vi "BG-corr-eventSD.vi"(1 "Single":bool, 2 "cluster in":T1={"Kinetics"=[], "Spectrum"=[], "Experiments groups"=[], "GRAPH EXPERIMENTAL DATA"=[], "error out"={"status"=FALSE, "code"=0, "source"=""}, "group"=0, "exp selected"=0, "# exp"=0, "kinetics plot names"=[], "spectra plot names"=[], "FromToWave"={"FromWave"=0.0, "ToWave"=0.0}, "Laser shutter task"="", "Accelerator task"="", "Motor task"="", "GRAPH EXPERIMENTAL DATA ref"=refnum, "timedelays"=[0.0, 0.0, 0.0, 0.0, 0.0, 0.0, 0.0, 0.06019061100911815, 0.0521779104562645, 0.045231877429679615, 0.03921051490799832, 0.033990728811568754, 0.029465811603150715, 0.025543260876973825, 0.02214288834180205, 0.01919518054014414, 0.016639877791965713, 0.014424742312398925, 0.012504490320209958, 0.010839866306230088, 0.009396840537117498, 0.008145913389103785, 0.00706151229029317, 0.006121468943269439, 0.005306566140927374, 0.004600144911132549, 0.003987763959109073, 0.0034569044455719407, 0.00299671406541447, 0.0025977851951783253, 0.0022519625739982996, 0.00195217658646366, 0.0016922987392150965, 0.0014670163768006634, 0.0012717240756200802, 0.0011024294957352762, 0.0009556717658856477, 0.0008284507332614981, 0.0007181656316962257, 0.0006225619144775864, 0.0005396851648867825, 0.00046784114226338394, 0.0004055611468220084, 0.0003515719951773376, 0.00030476999279031153, 0.00026419837125694315, 0.00022902772919263772, 0.0001985390768670671, 0.0001721091379728629, 0.00014919760805372974, 0.00012933610911736794], "wavelengths"=[0.0, 0.0, 0.0, 0.0, 0.0, 0.0, 0.0, 0.06019061100911815, 0.0521779104562645, 0.045231877429679615, 0.03921051490799832, 0.033990728811568754, 0.029465811603150715, 0.025543260876973825, 0.02214288834180205, 0.01919518054014414, 0.016639877791965713, 0.014424742312398925, 0.012504490320209958, 0.010839866306230088, 0.009396840537117498, 0.008145913389103785, 0.00706151229029317, 0.006121468943269439, 0.005306566140927374, 0.004600144911132549, 0.003987763959109073, 0.0034569044455719407, 0.00299671406541447, 0.0025977851951783253, 0.0022519625739982996, 0.00195217658646366, 0.0016922987392150965, 0.0014670163768006634, 0.0012717240756200802, 0.0011024294957352762, 0.0009556717658856477, 0.0008284507332614981, 0.0007181656316962257, 0.0006225619144775864, 0.0005396851648867825, 0.00046784114226338394, 0.0004055611468220084, 0.0003515719951773376, 0.00030476999279031153, 0.00026419837125694315, 0.00022902772919263772, 0.0001985390768670671, 0.0001721091379728629, 0.00014919760805372974, 0.00012933610911736794], "Experiment"=refnum, "Commentaires exp"=refnum, "FromToDelay"={"FromDelay"=0.0, "ToDelay"=0.0}}, 3 "Update graphs of exp":refnum<user-event>, 4 "def pixel lower":dbl, 5 "def pixel upper":dbl) -> (0 "cluster out":T1={"Kinetics"=[], "Spectrum"=[], "Experiments groups"=[], "GRAPH EXPERIMENTAL DATA"=[], "error out"={"status"=FALSE, "code"=0, "source"=""}, "group"=0, "exp selected"=0, "# exp"=0, "kinetics plot names"=[], "spectra plot names"=[], "FromToWave"={"FromWave"=0.0, "ToWave"=0.0}, "Laser shutter task"="", "Accelerator task"="", "Motor task"="", "GRAPH EXPERIMENTAL DATA ref"=refnum, "timedelays"=[0.0, 0.0, 0.0, 0.0, 0.0, 0.0, 0.0, 0.06019061100911815, 0.0521779104562645, 0.045231877429679615, 0.03921051490799832, 0.033990728811568754, 0.029465811603150715, 0.025543260876973825, 0.02214288834180205, 0.01919518054014414, 0.016639877791965713, 0.014424742312398925, 0.012504490320209958, 0.010839866306230088, 0.009396840537117498, 0.008145913389103785, 0.00706151229029317, 0.006121468943269439, 0.005306566140927374, 0.004600144911132549, 0.003987763959109073, 0.0034569044455719407, 0.00299671406541447, 0.0025977851951783253, 0.0022519625739982996, 0.00195217658646366, 0.0016922987392150965, 0.0014670163768006634, 0.0012717240756200802, 0.0011024294957352762, 0.0009556717658856477, 0.0008284507332614981, 0.0007181656316962257, 0.0006225619144775864, 0.0005396851648867825, 0.00046784114226338394, 0.0004055611468220084, 0.0003515719951773376, 0.00030476999279031153, 0.00026419837125694315, 0.00022902772919263772, 0.0001985390768670671, 0.0001721091379728629, 0.00014919760805372974, 0.00012933610911736794], "wavelengths"=[0.0, 0.0, 0.0, 0.0, 0.0, 0.0, 0.0, 0.06019061100911815, 0.0521779104562645, 0.045231877429679615, 0.03921051490799832, 0.033990728811568754, 0.029465811603150715, 0.025543260876973825, 0.02214288834180205, 0.01919518054014414, 0.016639877791965713, 0.014424742312398925, 0.012504490320209958, 0.010839866306230088, 0.009396840537117498, 0.008145913389103785, 0.00706151229029317, 0.006121468943269439, 0.005306566140927374, 0.004600144911132549, 0.003987763959109073, 0.0034569044455719407, 0.00299671406541447, 0.0025977851951783253, 0.0022519625739982996, 0.00195217658646366, 0.0016922987392150965, 0.0014670163768006634, 0.0012717240756200802, 0.0011024294957352762, 0.0009556717658856477, 0.0008284507332614981, 0.0007181656316962257, 0.0006225619144775864, 0.0005396851648867825, 0.00046784114226338394, 0.0004055611468220084, 0.0003515719951773376, 0.00030476999279031153, 0.00026419837125694315, 0.00022902772919263772, 0.0001985390768670671, 0.0001721091379728629, 0.00014919760805372974, 0.00012933610911736794], "Experiment"=refnum, "Commentaires exp"=refnum, "FromToDelay"={"FromDelay"=0.0, "ToDelay"=0.0}})   [LabVIEW 2015]
uses:
  controls/control-cluster.ctl
  Classes/Experiments_group.lvclass
types:
  T1 = typedef "control-cluster.ctl" = cluster{"Kinetics":cluster{"timedelay":dbl[], dbl[]}[], "Spectrum":cluster{"Unités abscisse":dbl[], dbl[]}[], "Experiments groups":refnum<class "Experiments_group.lvclass">[], "GRAPH EXPERIMENTAL DATA":dbl[][], "error out":errorcluster, "group":i32, "exp selected":i32, "# exp":i32, "kinetics plot names":string[], "spectra plot names":string[], "FromToWave":cluster{"FromWave":dbl, "ToWave":dbl}, "Laser shutter task":refnum<k21>, "Accelerator task":refnum<k21>, "Motor task":refnum<k21>, "GRAPH EXPERIMENTAL DATA ref":refnum<vi>, "timedelays":dbl[], "wavelengths":dbl[], "Experiment":refnum<vi>, "Commentaires exp":refnum<vi>, "FromToDelay":cluster{"FromDelay":dbl, "ToDelay":dbl}}
  T2 = typedef "mylistbox.ctl" = i32[]
  T3 = cluster{bool, "Item Names":string[], "exp selected":i32}
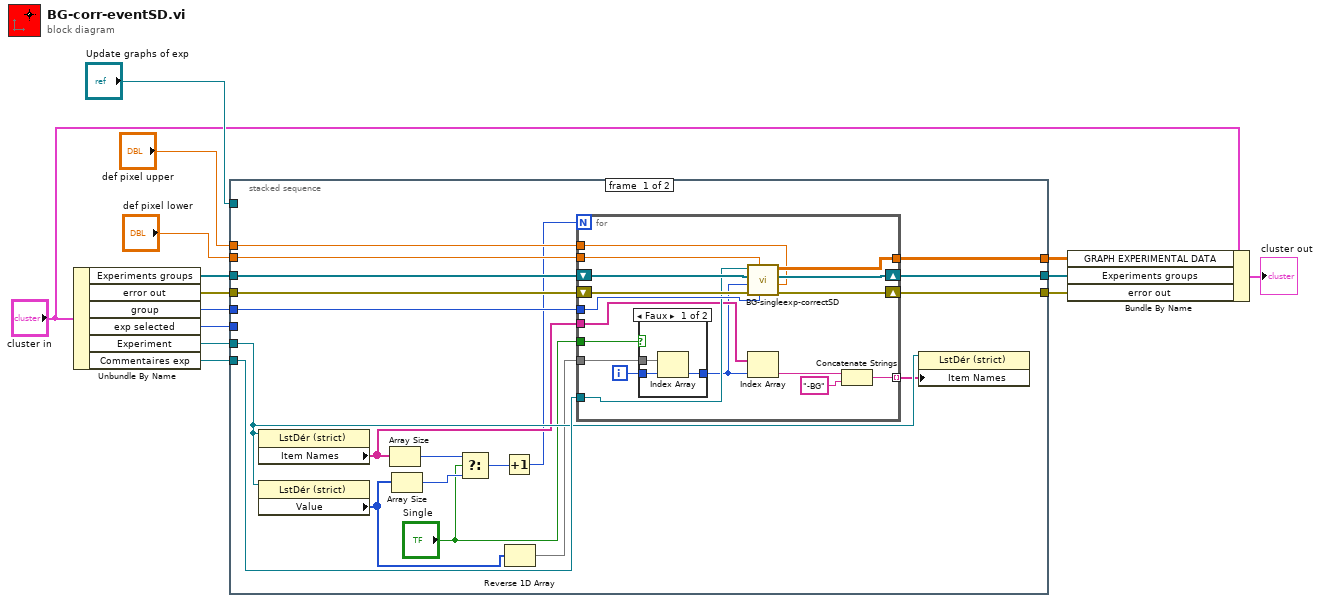
[diagram p0: block diagram]
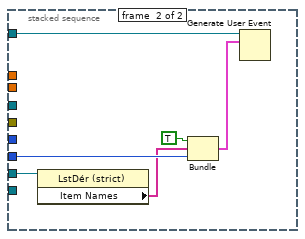
[diagram p3: hidden frame]
diagram:
  n1 = Unbundle By Name("cluster in") -> ("Experiments groups"=w8:refnum<class "Experiments_group.lvclass">[], "error out"=w7:errorcluster, "group"=w4:i32, "exp selected"=w5:i32, "Experiment"=w2:refnum<vi>, "Commentaires exp"=w1:refnum<vi>)
  n2 = stacked-sequence {
    tunnel: [w33 _] -> w9
    tunnel: w5 -> [_ w58]
    tunnel: w8 -> [w31 _]
    tunnel: w7 -> [w32 _]
    tunnel: [w25 _] -> w6
    tunnel: [w30 _] -> w3
    tunnel: "Update graphs of exp" -> [_ w59]
    tunnel: "def pixel lower" -> [w29 _]
    tunnel: "def pixel upper" -> [w28 _]
    tunnel: w4 -> [w27 _]
    tunnel: w1 -> [w26 _]
    tunnel: w2 -> [w24 w57]
    frame #0 {
      n3 = property on="Property Node" class="LstDér (strict)"(reference=w24) -> ("Item Names"=w17:string[])  [unwired: 1 in, 2 out]
      n4 = property class="LstDér (strict)"(reference=w24) -> ("Value"=w20:T2)  [unwired: 1 in, 2 out]
      n5 = Array Size(array=w17) -> (size(s)=w16:i32)
      n6 = Array Size(array=w20) -> (size(s)=w19:i32)
      n7 = Select(t=w16, s="Single", f=w19) -> (s? t:f=w22:i32)
      n8 = Increment(x=w22) -> (x+1=w15:i32)
      n9 = Reverse 1D Array(array=w20) -> (reversed array=w21:T2)
      n10 = for {
        N: w15 -> [_]
        tunnel: [w47] -> w30
        tunnel: w29 -> [w46]
        tunnel: w28 -> [w45]
        tunnel: w27 -> [w44]
        tunnel: w26 -> [w43]
        shift-right: [w42] -> w25
        shift-left: w32 -> [w49]
        tunnel: w21 -> [w35]
        tunnel: w17 -> [w39]
        tunnel: [w38] -> w23 mode=indexing
        shift-right: [w50] -> w33
        shift-left: w31 -> [w48]
        tunnel: "Single" -> [w37]
        i -> [w36]
        n11 = case shown="Faux" w37 {
          tunnel: w36 -> [w51 w54]
          tunnel: [w52 w54] -> w34
          tunnel: w35 -> [w53 _]
          frame False {
            n12 = Index Array(array=w53, index=w51) -> (element=w52:i32)
          }
          frame True {
          }
        }
        n13 = call "BG-singleexp-correctSD.vi"("def pixel upper"=w45, "group"=w44, "def pixel lower"=w46, "error in (no error)"=w49, "exp selected"=w34, "Experiments groups"=w48, "Commentaires"=w43) -> ("error out"=w42:errorcluster, "Experiments groups out"=w50:refnum<class "Experiments_group.lvclass">[], "Array"=w47:dbl[][])
        n14 = Index Array(array=w39, index=w34) -> (element=w40:string)
        n15 = Concatenate Strings(w40, "-BG" ("string")) -> (w38:string)
      }
      n16 = property on="Property Node" class="LstDér (strict)"(reference=w24, "Item Names"=w23) -> ()  [unwired: 1 in, 2 out]
    }
    frame #1 {
      n17 = property on="Property Node" class="LstDér (strict)"(reference=w57) -> ("Item Names"=w56:string[])  [unwired: 1 in, 2 out]
      n18 = Bundle(TRUE, "Item Names"=w56, "exp selected"=w58) -> (w55:T3)  [unwired: 1 in]
      n19 = Generate User Event(user event=w59, event data cluster=w55) -> ()  [unwired: 2 in, 2 out]
    }
  }
  n20 = Bundle By Name(cluster="cluster in", "GRAPH EXPERIMENTAL DATA"=w3, "Experiments groups"=w9, "error out"=w6) -> (→"cluster out":T1)
